vi "ConfigDevice.vi"(8 "error in (no error)":errorcluster, 11 "NHRDCPower in":refnum<class "NHRDCPower.lvclass">) -> (0 "error out":errorcluster, 3 "NHRDCPower out":refnum<class "NHRDCPower.lvclass">)   [LabVIEW 2018, in "AcPwrPlugins.lvlib" / "NHRDCPower.lvclass"]
doc: "This VI configures all the properties set by the user through the INI file or the Properties Dialog box."
uses:
  NHRDCPower.lvclass
  <instrlib>/NHRDCPowerModule/NHRDCPowerModule/NHRDCPowerModule.lvlib
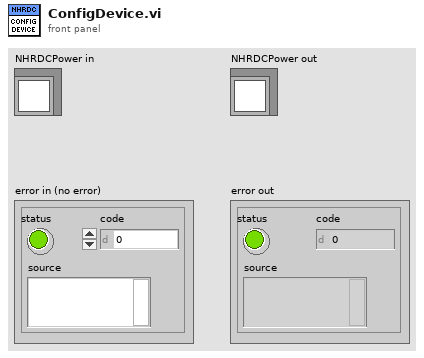
[diagram p1: front panel]
types:
  T1 = typedef "AcPwrPlugins.lvlib/NHRDCPower.lvclass/Device(s)Settings.ctl" = cluster{"Handle":string, "Name":string, "id query (Yes)":bool, "reset device (Yes)":bool, "Connected":bool, "Voltage Range (V)":dbl[], "Timing":cluster{"TimingOn":enum16{""}, "Hours":u32, "Minutes":u32, "Seconds":dbl, "CutoffVoltage":dbl}, "SlewRate":cluster{"Set Voltage Rate V/S":sgl, "Set Current Rate A/S":sgl, "Set Resistance Rate R/S":sgl, "Set Power Rate W/S":sgl}, "OutputSettings":cluster{"operating state (Off)":i32, "Voltage (V)":sgl, "Current (A)":sgl, "Resistance (Ohms)":sgl, "Power (W)":sgl, "Enable Voltage":bool, "Enable Current":bool, "Enable Resistance":bool, "Enable Power":bool, "Aperture Time (s)":sgl}, "Initial Battery Detect Voltage (0)":dbl, "SafetySettings":cluster{"SetWatchDog":bool, "Voltage (V)":sgl, "Current (A)":sgl, "Power (W)":sgl, "Voltage Delay (s)":sgl, "Current Delay (s)":sgl, "Power Delay (s)":sgl}, "Options String":string}[]
  T2 = cluster{"SetWatchDog":bool, "Voltage (V)":sgl, "Current (A)":sgl, "Power (W)":sgl, "Voltage Delay (s)":sgl, "Current Delay (s)":sgl, "Power Delay (s)":sgl}
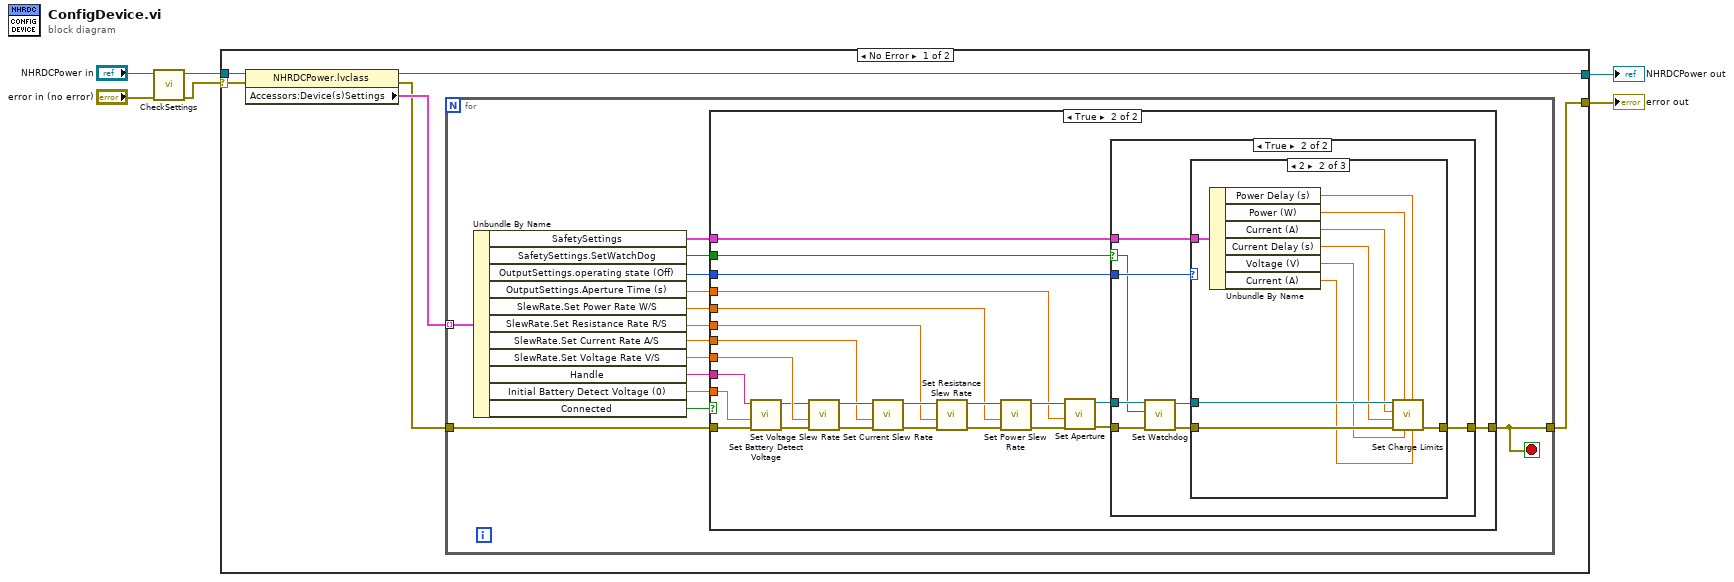
[diagram p0: block diagram]
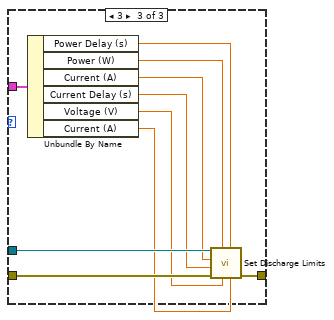
[diagram p5: hidden frame]
diagram:
  n1 = call-dynamic "CheckSettings.vi"("error in (no error)"="error in (no error)", "NHRDCPower in"="NHRDCPower in") -> ("error out"=w1:errorcluster, "NHRDCPower out"=w3:refnum<class "NHRDCPower.lvclass">)  [unwired: 8 in]
  n2 = case shown="No Error" w1 {
    selector: w1 -> [w11 w82]
    tunnel: w3 -> [w12 w83]
    tunnel: [w10 w83] -> w6
    tunnel: [w7 w82] -> w5
    frame No Error {
      n3 = property class="NHRDCPower.lvclass"(reference=w12, error in=w11) -> (reference out=w10:refnum<class "NHRDCPower.lvclass">, error out=w8:errorcluster, "Accessors:Device(s)Settings"=w9:T1)
      n4 = for {
        tunnel: w9 -> [w26] mode=indexing
        tunnel: w8 -> [w25]
        tunnel: [w20] -> w7
        stop <- w20 stop-if-true
        n5 = Unbundle By Name(w26) -> ("SafetySettings"=w15:T2, "SafetySettings.SetWatchDog"=w14:bool, "OutputSettings.operating state (Off)"=w23:i32, "OutputSettings.Aperture Time (s)"=w24:sgl, "SlewRate.Set Power Rate W/S"=w22:sgl, "SlewRate.Set Resistance Rate R/S"=w21:sgl, "SlewRate.Set Current Rate A/S"=w16:sgl, "SlewRate.Set Voltage Rate V/S"=w17:sgl, "Handle"=w18:string, "Initial Battery Detect Voltage (0)"=w13:dbl, "Connected"=w19:bool)
        n6 = case shown="True" w19 {
          tunnel: w25 -> [w27 w51]
          tunnel: w24 -> [_ w35]
          tunnel: w23 -> [_ w34]
          tunnel: w22 -> [_ w36]
          tunnel: w21 -> [_ w37]
          tunnel: [w27 w42] -> w20
          tunnel: w18 -> [_ w30]
          tunnel: w17 -> [_ w39]
          tunnel: w16 -> [_ w38]
          tunnel: w15 -> [_ w33]
          tunnel: w14 -> [_ w32]
          tunnel: w13 -> [_ w28]
          frame False {
          }
          frame True {
            n7 = call <instrlib>:"Set Battery Detect Voltage.vi"("error in (no error)"=w51, "minimum voltage (4.0)"=w28, "instrument handle"=w30) -> ("error out"=w31:errorcluster, "instrument handle out"=w29:refnum<visa-resource-name>)  [unwired: 7 in]
            n8 = call <instrlib>:"Set Voltage Slew Rate.vi"("error in (no error)"=w31, "voltage slew rate (0.0)"=w39, "instrument handle"=w29) -> ("error out"=w50:errorcluster, "instrument handle out"=w46:refnum<visa-resource-name>)  [unwired: 7 in]
            n9 = call <instrlib>:"Set Current Slew Rate.vi"("error in (no error)"=w50, "current slew rate (0.0)"=w38, "instrument handle"=w46) -> ("error out"=w49:errorcluster, "instrument handle out"=w45:refnum<visa-resource-name>)  [unwired: 7 in]
            n10 = call <instrlib>:"Set Resistance Slew Rate.vi"("error in (no error)"=w49, "resistance slew rate (0.0)"=w37, "instrument handle"=w45) -> ("error out"=w48:errorcluster, "instrument handle out"=w44:refnum<visa-resource-name>)  [unwired: 7 in]
            n11 = call <instrlib>:"Set Power Slew Rate.vi"("error in (no error)"=w48, "power slew rate (0.0)"=w36, "instrument handle"=w44) -> ("error out"=w47:errorcluster, "instrument handle out"=w43:refnum<visa-resource-name>)  [unwired: 7 in]
            n12 = call <instrlib>:"Set Aperture.vi"("error in (no error)"=w47, "aperture (0.0)"=w35, "instrument handle"=w43) -> ("error out"=w41:errorcluster, "instrument handle out"=w40:refnum<visa-resource-name>)  [unwired: 7 in]
            n13 = case shown="True" w32 {
              selector: w32 -> [_ w54]
              tunnel: w41 -> [w52 w60]
              tunnel: [w52 w59] -> w42
              tunnel: w40 -> [_ w57]
              tunnel: w34 -> [_ w55]
              tunnel: w33 -> [_ w53]
              frame False {
              }
              frame True {
                n14 = call <instrlib>:"Set Watchdog.vi"("error in (no error)"=w60, "watchdog"=w54, "instrument handle"=w57) -> ("error out"=w58:errorcluster, "instrument handle out"=w56:refnum<visa-resource-name>)  [unwired: 7 in]
                n15 = case shown="2" w55 {
                  tunnel: w58 -> [w61 w71 w81]
                  tunnel: [w61 w70 w80] -> w59
                  tunnel: w56 -> [_ w69 w79]
                  tunnel: w53 -> [_ w62 w72]
                  frame 0, Default {
                  }
                  frame 2 {
                    n16 = Unbundle By Name(w62) -> ("Power Delay (s)"=w68:sgl, "Power (W)"=w67:sgl, "Current (A)"=w66:sgl, "Current Delay (s)"=w65:sgl, "Voltage (V)"=w64:sgl, "Current (A)"=w63:sgl)
                    n17 = call <instrlib>:"Set Charge Limits.vi"("voltage delay (0.0)"=w63, "power delay (0.0)"=w68, "voltage max"=w64, "power"=w67, "error in (no error)"=w71, "current delay (0.0)"=w65, "current"=w66, "instrument handle"=w69) -> ("error out"=w70:errorcluster)  [unwired: 2 in, 1 out]
                  }
                  frame 3 {
                    n18 = Unbundle By Name(w72) -> ("Power Delay (s)"=w78:sgl, "Power (W)"=w77:sgl, "Current (A)"=w76:sgl, "Current Delay (s)"=w75:sgl, "Voltage (V)"=w74:sgl, "Current (A)"=w73:sgl)
                    n19 = call <instrlib>:"Set Discharge Limits.vi"("voltage delay (0.0)"=w73, "power delay (0.0)"=w78, "voltage min"=w74, "power"=w77, "error in (no error)"=w81, "current delay (0.0)"=w75, "current"=w76, "instrument handle"=w79) -> ("error out"=w80:errorcluster)  [unwired: 2 in, 1 out]
                  }
                }
              }
            }
          }
        }
      }
    }
    frame Error {
    }
  }
  "error out" <- w5
  "NHRDCPower out" <- w6
